vi "WriteData (WFM).vi"(6 "value index (0)":u64, 7 "WFM":waveform(dbl), 8 "error in (no error)":errorcluster, 9 "channel index (0)":u32, 10 "operation (0: create)":T2(ring)=enum."Create", 11 "Excel refnum":T1) -> (0 "error out":errorcluster, 3 "Excel refnum out":T1)   [LabVIEW 2020, in "NI_ExcelFile.lvlib"]
uses:
  <vilib>/express/express shared/NI_ExcelFile/NI_ExcelFile.lvlib
  <vilib>/express/express shared/NI_ExcelFile/Ctrls/ExcelRefnum.ctl
  <vilib>/express/express shared/NI_ExcelFile/Ctrls/MainData.ctl
  <vilib>/express/express shared/NI_ExcelFile/Ctrls/StreamMode.ctl
  <vilib>/express/express shared/NI_ExcelFile/Ctrls/TimeColumnMode.ctl
  <vilib>/express/express shared/NI_ExcelFile/Ctrls/FileAttribute.ctl
  <vilib>/express/express shared/NI_ExcelFile/Ctrls/Columns.ctl
  <vilib>/express/express shared/NI_ExcelFile/Ctrls/ColumnInfo.ctl
  <vilib>/express/express shared/NI_ExcelFile/Ctrls/DataType.ctl
  <vilib>/express/express shared/NI_ExcelFile/Ctrls/wd_recordInfo.ctl
  <vilib>/express/express shared/NI_ExcelFile/Ctrls/disk_TemplateFile.ctl
  <vilib>/express/express shared/NI_ExcelFile/Ctrls/meta_file.ctl
  <vilib>/express/express shared/NI_ExcelFile/Ctrls/meta_Block.ctl
  <vilib>/express/express shared/NI_ExcelFile/Ctrls/meta_BlockType.ctl
  <vilib>/express/express shared/NI_ExcelFile/SubVIs/utilities_addTime.vi
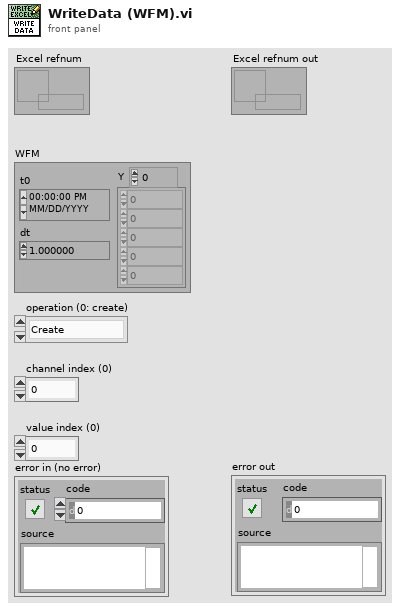
[diagram p1: front panel]
types:
  T1 = typedef "NI_ExcelFile.lvlib/ExcelRefnum.ctl" = refnum<data-value>
  T2 = enum16{"Append values", "Create", "Replace values at index", "Replace all values"}
  T3 = typedef "NI_ExcelFile.lvlib/DataType.ctl" = enum16{"DDT", "WFM", "Array of STR", "Array of DBL", "Array of I8", "Array of I16", "Array of I32", "Array of I64", "Array of SGL", "Array of U8", "Array of U16", "Array of U32", "Array of U64", "Array of Time"}
  T4 = typedef "NI_ExcelFile.lvlib/MainData.ctl" = cluster{"TargetFile":path, "StreamMode":T5, "Append?":bool, "ChunkSize":u64, "TimeColumnMode":T6, "TimestampFormat":string, "AbsoluteTime?":bool, "FileAttribute ":T7, "Column":T8, "FileRef":refnum<k1>, "MemoryRef":refnum<data-value>[], "RecordInfo":T10[], " ChannelPreviousInfo":u32[], "ChannelFirstRecord":u32[], "PredefinedFormattedValueLength":i64, "DiskTemplate":T11}
  T5 = typedef "NI_ExcelFile.lvlib/StreamMode.ctl" = enum16{"File", "Memory"}
  T6 = typedef "NI_ExcelFile.lvlib/TimeColumnMode.ctl" = enum16{"Empty", "OnePerCh", "One"}
  T7 = typedef "NI_ExcelFile.lvlib/FileAttribute.ctl" = cluster{"Creator":string, "Title":string, "SheetName":string}
  T8 = typedef "NI_ExcelFile.lvlib/Columns.ctl" = T9[]
  T9 = typedef "NI_ExcelFile.lvlib/ColumnInfo.ctl" = cluster{"Header":string, "Format":string, "DataType":T3, "Length":u64}
  T10 = typedef "NI_ExcelFile.lvlib/wd_recordInfo.ctl" = cluster{"ChannelIndex":u32, "StartIndex":u64, "Length":u64, "Previous":i32, "Next":i32}
  T11 = typedef "NI_ExcelFile.lvlib/disk_TemplateFile.ctl" = cluster{"XMLRef":refnum<file>[], "ZipPath":path, "MetaFile":T12, "TempFolder":path}
  T12 = typedef "NI_ExcelFile.lvlib/meta_file.ctl" = cluster{"Ref":refnum<file>, "NextRow":i32, "NextPosition":i64, "Block":T13[]}
  T13 = typedef "NI_ExcelFile.lvlib/meta_Block.ctl" = cluster{"Version":u16, "Type":T14, "Length":i32, "Data":string}
  T14 = typedef "NI_ExcelFile.lvlib/meta_BlockType.ctl" = enum16{"NITag", "File", "Column"}
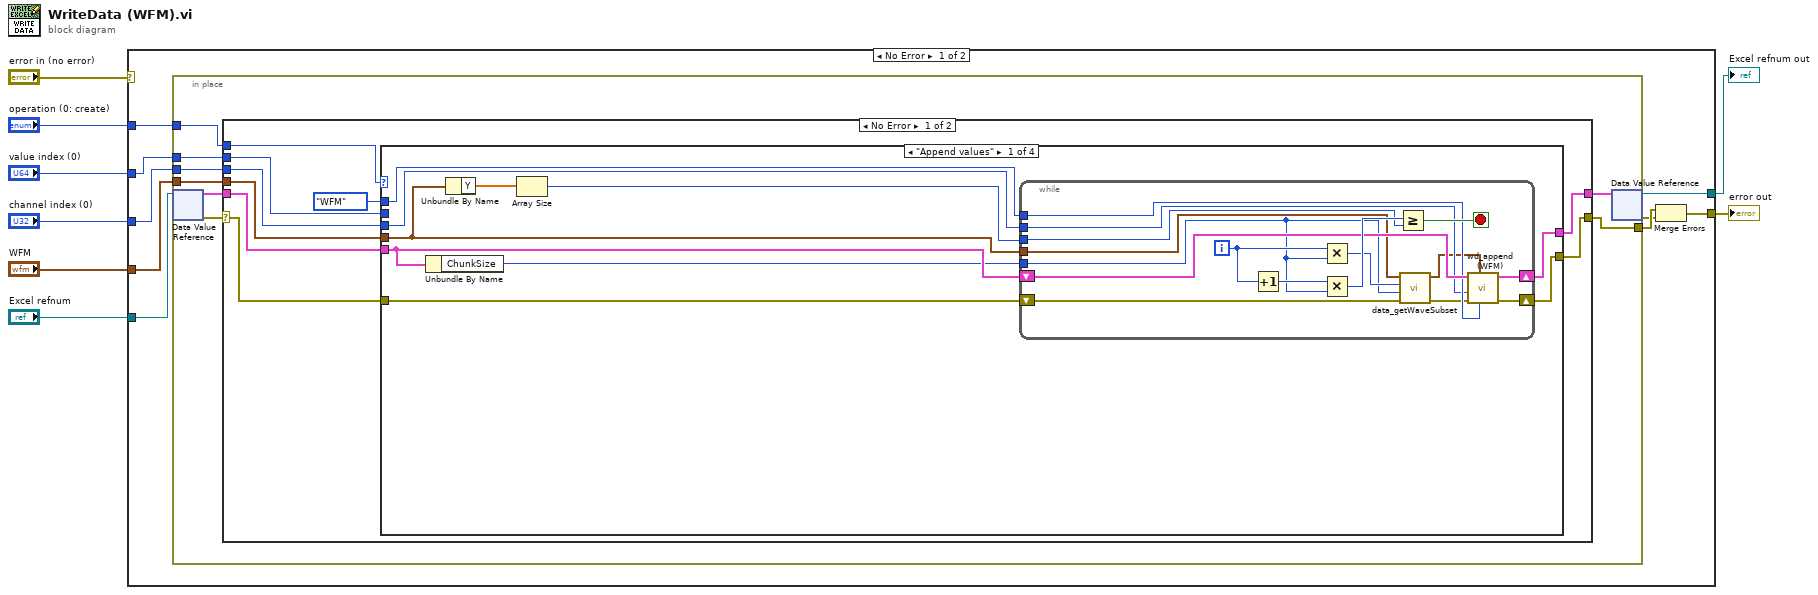
[diagram p0: block diagram]
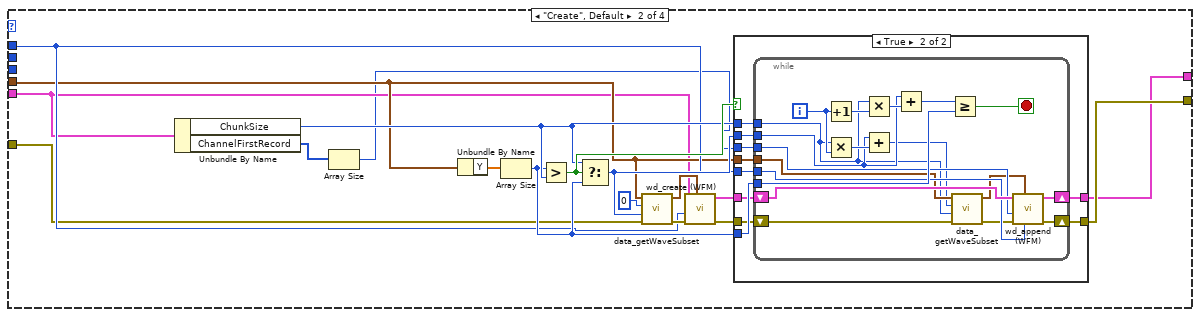
[diagram p2: hidden frame]
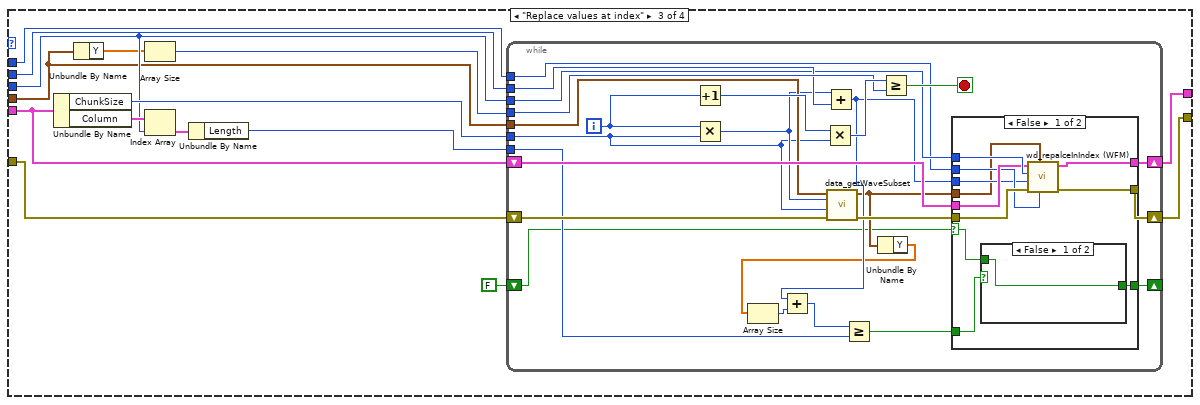
[diagram p4: hidden frame]
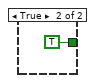
[diagram p5: hidden frame]
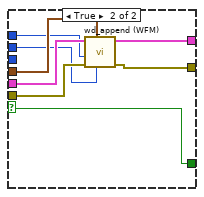
[diagram p6: hidden frame]
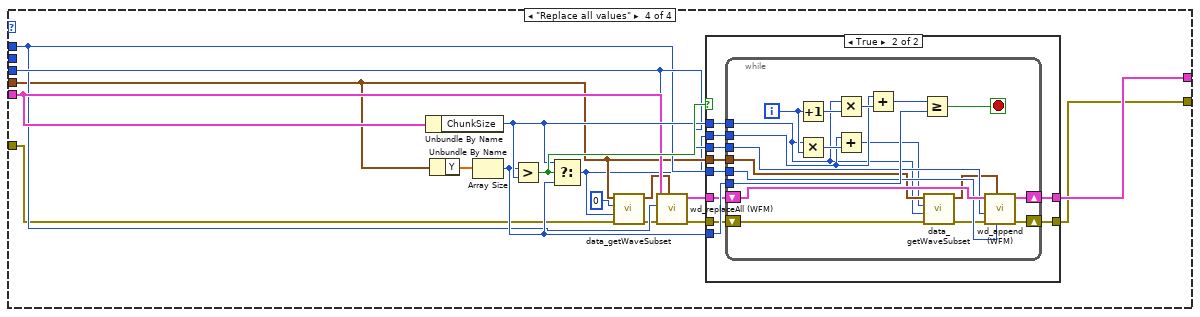
[diagram p7: hidden frame]
diagram:
  n1 = case shown="No Error" "error in (no error)" {
    selector: "error in (no error)" -> [_ w222]
    tunnel: "WFM" -> [w14 _]
    tunnel: [w9 w222] -> w2
    tunnel: "Excel refnum" -> [w17 w221]
    tunnel: [w16 w221] -> w3
    tunnel: "operation (0: create)" -> [w15 _]
    tunnel: "channel index (0)" -> [w13 _]
    tunnel: "value index (0)" -> [w12 _]
    frame No Error {
      n2 = in-place {
        in-place-border: w15 -> [w23]
        in-place-border: w14 -> [w22]
        in-place-border: w13 -> [w21]
        in-place-border: [w20] -> w11
        in-place-border: w12 -> [w19]
        n3 = in-place-dvr #1(w17) -> (w25:T4, w18:errorcluster)
        n4 = case shown="No Error" w18 {
          selector: w18 -> [w26 w219]
          tunnel: w25 -> [w34 w220]
          tunnel: [w33 w220] -> w24
          tunnel: w23 -> [w32 _]
          tunnel: w22 -> [w31 _]
          tunnel: w21 -> [w30 _]
          tunnel: [w29 w219] -> w20
          tunnel: w19 -> [w28 _]
          frame No Error {
            n5 = case shown="\"Append values\"" w32 {
              tunnel: w34 -> [w41 w66 w122 w182]
              tunnel: [w38 w63 w119 w179] -> w33
              tunnel: w31 -> [w36 w67 w113 w175]
              tunnel: w30 -> [w39 _ w116 w181]
              tunnel: w26 -> [w42 w65 w111 w172]
              tunnel: [w37 w64 w118 w178] -> w29
              tunnel: w28 -> [_ _ w120 _]
              tunnel: DataType."WFM" ("new element/subarray") -> [w43 w68 w121 w180]
              frame "Append values" {
                n6 = Unbundle By Name(w41) -> ("ChunkSize"=w40:u64)
                n7 = Unbundle By Name(w36) -> ("Y"=w35:dbl[])
                n8 = Array Size(array=w35) -> (size(s)=w44:i32)
                n9 = while {
                  tunnel: w40 -> [w48]
                  tunnel: w44 -> [w58]
                  tunnel: w43 -> [w55]
                  tunnel: w36 -> [w50]
                  shift-right: [w52] -> w38
                  shift-left: w41 -> [w56]
                  shift-right: [w53] -> w37
                  shift-left: w42 -> [w46]
                  tunnel: w39 -> [w51]
                  i -> [w54]
                  stop <- w57 stop-if-true
                  n10 = Increment(x=w54) -> (x+1=w60:i32)
                  n11 = Multiply(x=w54, y=w48) -> (x*y=w49:u64)
                  n12 = Multiply(x=w60, y=w48) -> (x*y=w59:u64)
                  n13 = Greater Or Equal?(x=w59, y=w58) -> (x >= y?=w57:bool)
                  n14 = call <vilib>:"data_getWaveSubset.vi"("error in (no error)"=w46, "length"=w48, "index"=w49, "Waveform"=w50) -> ("error out"=w45:errorcluster, "Waveform out"=w47:waveform(dbl))  [unwired: 6 in]
                  n15 = call <vilib>:"wd_append (WFM).vi"("data type"=w55, "Waveform"=w47, "error in (no error)"=w45, "channel index"=w51, "meta in"=w56) -> ("error out"=w53:errorcluster, "meta out"=w52:T4)  [unwired: 5 in]
                }
              }
              frame "Create", Default {
                n16 = Unbundle By Name(w66) -> ("ChunkSize"=w75:u64, "ChannelFirstRecord"=w62:u32[])
                n17 = Array Size(array=w62) -> (size(s)=w61:i32)
                n18 = Unbundle By Name(w67) -> ("Y"=w73:dbl[])
                n19 = Array Size(array=w73) -> (size(s)=w74:i32)
                n20 = Greater?(x=w74, y=w75) -> (0:w78:bool)
                n21 = Select(t=w75, s=w78, f=w74) -> (s? t:f=w71:u64)
                n22 = call <vilib>:"data_getWaveSubset.vi"("error in (no error)"=w65, "length"=w71, "index"=u64 0 ("start samples/time"), "Waveform"=w67) -> ("error out"=w69:errorcluster, "Waveform out"=w72:waveform(dbl))  [unwired: 6 in]
                n23 = call <vilib>:"wd_create (WFM).vi"("WFM"=w72, "error in (no error)"=w69, "data type"=w68, "meta in"=w66) -> ("error out"=w76:errorcluster, "meta out"=w77:T4)  [unwired: 6 in]
                n24 = case shown="True" w78 {
                  tunnel: [w80 w82] -> w63
                  tunnel: w77 -> [w80 w86]
                  tunnel: [w79 w81] -> w64
                  tunnel: w76 -> [w79 w83]
                  tunnel: w75 -> [_ w90]
                  tunnel: w71 -> [_ w89]
                  tunnel: w74 -> [_ w88]
                  tunnel: w67 -> [_ w87]
                  tunnel: w61 -> [_ w85]
                  tunnel: w68 -> [_ w84]
                  frame False {
                  }
                  frame True {
                    n25 = while {
                      tunnel: w90 -> [w93]
                      tunnel: w89 -> [w102]
                      tunnel: w88 -> [w106]
                      tunnel: w87 -> [w95]
                      shift-right: [w100] -> w82
                      shift-left: w86 -> [w101]
                      tunnel: w85 -> [w99]
                      tunnel: w84 -> [w98]
                      shift-right: [w97] -> w81
                      shift-left: w83 -> [w92]
                      i -> [w104]
                      stop <- w105 stop-if-true
                      n26 = Increment(x=w104) -> (x+1=w109:i32)
                      n27 = Multiply(x=w93, y=w104) -> (x*y=w103:u64)
                      n28 = Multiply(x=w93, y=w109) -> (x*y=w108:u64)
                      n29 = Add(x=w102, y=w103) -> (x+y=w94:u64)
                      n30 = Add(x=w102, y=w108) -> (x+y=w107:u64)
                      n31 = Greater Or Equal?(x=w107, y=w106) -> (x >= y?=w105:bool)
                      n32 = call <vilib>:"data_getWaveSubset.vi"("error in (no error)"=w92, "length"=w93, "index"=w94, "Waveform"=w95) -> ("error out"=w91:errorcluster, "Waveform out"=w96:waveform(dbl))  [unwired: 6 in]
                      n33 = call <vilib>:"wd_append (WFM).vi"("data type"=w98, "Waveform"=w96, "error in (no error)"=w91, "channel index"=w99, "meta in"=w101) -> ("error out"=w97:errorcluster, "meta out"=w100:T4)  [unwired: 5 in]
                    }
                  }
                }
              }
              frame "Replace values at index" {
                n34 = Unbundle By Name(w122) -> ("ChunkSize"=w123:u64, "Column"=w117:T8)
                n35 = Unbundle By Name(w113) -> ("Y"=w112:dbl[])
                n36 = Array Size(array=w112) -> (size(s)=w124:i32)
                n37 = Index Array(array=w117, index=w116) -> (element=w115:T9)
                n38 = Unbundle By Name(w115) -> ("Length"=w114:u64)
                n39 = while {
                  tunnel: w123 -> [w136]
                  tunnel: w124 -> [w147]
                  tunnel: w121 -> [w141]
                  tunnel: w113 -> [w138]
                  shift-right: [w140] -> w119
                  shift-left: w122 -> [w142]
                  shift-right: [w139] -> w118
                  shift-left: w111 -> [w135]
                  tunnel: w116 -> [w143]
                  tunnel: w120 -> [w144]
                  tunnel: w114 -> [w131]
                  shift-right: [w125] -> _
                  shift-left: FALSE ("Append?") -> [w126]
                  i -> [w145]
                  stop <- w146 stop-if-true
                  n40 = Increment(x=w145) -> (x+1=w149:i32)
                  n41 = Multiply(x=w145, y=w136) -> (x*y=w137:u64)
                  n42 = Multiply(x=w149, y=w136) -> (x*y=w148:u64)
                  n43 = Add(x=w137, y=w144) -> (x+y=w130:u64)
                  n44 = call <vilib>:"data_getWaveSubset.vi"("error in (no error)"=w135, "length"=w136, "index"=w137, "Waveform"=w138) -> ("error out"=w134:errorcluster, "Waveform out"=w129:waveform(dbl))  [unwired: 6 in]
                  n45 = Unbundle By Name(w129) -> ("Y"=w128:dbl[])
                  n46 = Array Size(array=w128) -> (size(s)=w132:i32)
                  n47 = Add(x=w130, y=w132) -> (x+y=w133:u64)
                  n48 = Greater Or Equal?(x=w133, y=w131) -> (x >= y?=w127:bool)
                  n49 = Greater Or Equal?(x=w148, y=w147) -> (x >= y?=w146:bool)
                  n50 = case shown="False" w126 {
                    selector: w126 -> [w151 w163]
                    tunnel: w143 -> [w160 w168]
                    tunnel: w142 -> [w159 w169]
                    tunnel: w129 -> [w153 w170]
                    tunnel: w134 -> [w158 w167]
                    tunnel: w130 -> [w154 _]
                    tunnel: w141 -> [w157 w166]
                    tunnel: [w156 w165] -> w140
                    tunnel: [w155 w164] -> w139
                    tunnel: w127 -> [w152 _]
                    tunnel: [w150 w163] -> w125
                    frame False {
                      n51 = case shown="False" w152 {
                        tunnel: w151 -> [w161 _]
                        tunnel: [w161 TRUE] -> w150
                        frame False {
                        }
                        frame True {
                        }
                      }
                      n52 = call <vilib>:"wd_repalceInIndex (WFM).vi"("data type"=w157, "WFM"=w153, "error in (no error)"=w158, "value index"=w154, "channel index"=w160, "meta in"=w159) -> ("error out"=w155:errorcluster, "meta out"=w156:T4)  [unwired: 4 in]
                    }
                    frame True {
                      n53 = call <vilib>:"wd_append (WFM).vi"("data type"=w166, "Waveform"=w170, "error in (no error)"=w167, "channel index"=w168, "meta in"=w169) -> ("error out"=w164:errorcluster, "meta out"=w165:T4)  [unwired: 5 in]
                    }
                  }
                }
              }
              frame "Replace all values" {
                n54 = Unbundle By Name(w182) -> ("ChunkSize"=w184:u64)
                n55 = Unbundle By Name(w175) -> ("Y"=w177:dbl[])
                n56 = Array Size(array=w177) -> (size(s)=w183:i32)
                n57 = Greater?(x=w183, y=w184) -> (0:w187:bool)
                n58 = Select(t=w184, s=w187, f=w183) -> (s? t:f=w174:u64)
                n59 = call <vilib>:"data_getWaveSubset.vi"("error in (no error)"=w172, "length"=w174, "index"=u64 0 ("start samples/time"), "Waveform"=w175) -> ("error out"=w171:errorcluster, "Waveform out"=w176:waveform(dbl))  [unwired: 6 in]
                n60 = call <vilib>:"wd_replaceAll (WFM).vi"("WFM"=w176, "error in (no error)"=w171, "channel index"=w181, "data type"=w180, "meta in"=w182) -> ("error out"=w185:errorcluster, "meta out"=w186:T4)  [unwired: 5 in]
                n61 = case shown="True" w187 {
                  tunnel: [w189 w191] -> w179
                  tunnel: w186 -> [w189 w195]
                  tunnel: [w188 w190] -> w178
                  tunnel: w185 -> [w188 w192]
                  tunnel: w184 -> [_ w199]
                  tunnel: w174 -> [_ w198]
                  tunnel: w183 -> [_ w197]
                  tunnel: w175 -> [_ w196]
                  tunnel: w181 -> [_ w194]
                  tunnel: w180 -> [_ w193]
                  frame False {
                  }
                  frame True {
                    n62 = while {
                      tunnel: w199 -> [w202]
                      tunnel: w198 -> [w211]
                      tunnel: w197 -> [w215]
                      tunnel: w196 -> [w204]
                      shift-right: [w209] -> w191
                      shift-left: w195 -> [w210]
                      tunnel: w194 -> [w208]
                      tunnel: w193 -> [w207]
                      shift-right: [w206] -> w190
                      shift-left: w192 -> [w201]
                      i -> [w213]
                      stop <- w214 stop-if-true
                      n63 = Increment(x=w213) -> (x+1=w218:i32)
                      n64 = Multiply(x=w202, y=w213) -> (x*y=w212:u64)
                      n65 = Multiply(x=w202, y=w218) -> (x*y=w217:u64)
                      n66 = Add(x=w211, y=w212) -> (x+y=w203:u64)
                      n67 = Add(x=w211, y=w217) -> (x+y=w216:u64)
                      n68 = Greater Or Equal?(x=w216, y=w215) -> (x >= y?=w214:bool)
                      n69 = call <vilib>:"data_getWaveSubset.vi"("error in (no error)"=w201, "length"=w202, "index"=w203, "Waveform"=w204) -> ("error out"=w200:errorcluster, "Waveform out"=w205:waveform(dbl))  [unwired: 6 in]
                      n70 = call <vilib>:"wd_append (WFM).vi"("data type"=w207, "Waveform"=w205, "error in (no error)"=w200, "channel index"=w208, "meta in"=w210) -> ("error out"=w206:errorcluster, "meta out"=w209:T4)  [unwired: 5 in]
                    }
                  }
                }
              }
            }
          }
          frame Error {
          }
        }
        n71 = in-place-dvr #1(w24) -> (w16:T1, w10:errorcluster)
      }
      n72 = Merge Errors(w11, w10) -> (w9:errorcluster)
    }
    frame Error {
    }
  }
  "Excel refnum out" <- w3
  "error out" <- w2
